vi "svl_Peak Resampled Level (N Ch).vi"(8 "error in (no error)":errorcluster, 9 "processing state":T1(ring), 11 "scaled even angle signals [EU]":T2(array[cluster]) {"even angle signal" format="%.2f"; "dr" format="%.2f"; "r0" format="%.2f"}) -> (0 "error out":errorcluster, 3 "peak levels":dbl[](array[numeric]) format="%.2f")   [LabVIEW 2017]
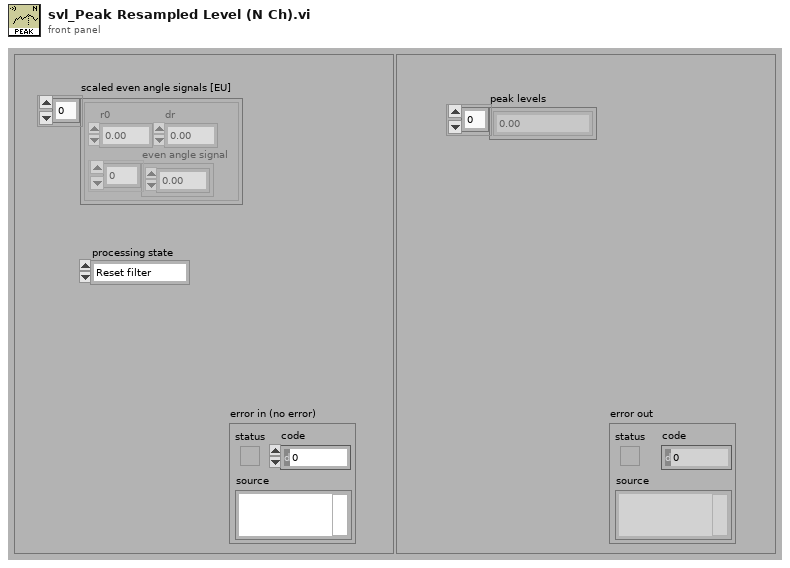
[diagram p1: front panel]
types:
  T1 = enum16{"Reset filter", "Restart averaging", "Continue processing"}
  T2 = cluster{"r0":dbl, "dr":dbl, "even angle signal":dbl[]}[]
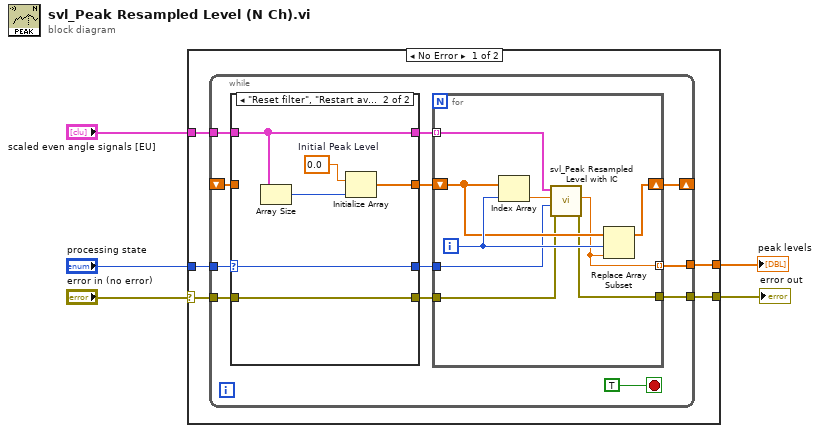
[diagram p0: block diagram]
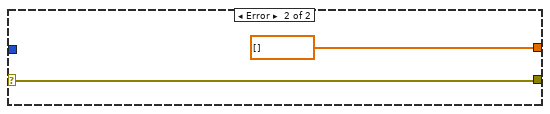
[diagram p3: hidden frame]
diagram:
  n1 = case shown="No Error" "error in (no error)" {
    selector: "error in (no error)" -> [w7 w43]
    tunnel: "processing state" -> [w10 _]
    tunnel: "scaled even angle signals [EU]" -> [w9 _]
    tunnel: [w8 dbl[] []] -> w3
    tunnel: [w6 w43] -> w1
    frame No Error {
      n2 = while {
        tunnel: [w13] -> w6
        tunnel: w7 -> [w12]
        tunnel: [w16] -> w8
        shift-left: _ -> [w18]
        shift-right: [w21] -> _
        tunnel: w9 -> [w15]
        tunnel: w10 -> [w20]
        stop <- TRUE stop-if-true
        n3 = case shown="\"Reset filter\", \"Restart averaging\"" w20 {
          selector: w20 -> [w26 w32]
          tunnel: [w26 w32] -> w19
          tunnel: w18 -> [w25 _]
          tunnel: [w25 w31] -> w17
          tunnel: w15 -> [w24 w30]
          tunnel: [w24 w30] -> w14
          tunnel: w12 -> [w23 w29]
          tunnel: [w23 w29] -> w11
          frame "Continue processing", Default {
          }
          frame "Reset filter", "Restart averaging" {
            w28 = 0.0  # Initial Peak Level
            n4 = Array Size(array=w30) -> (size(s)=w27:i32)
            n5 = Initialize Array(w28, w27) -> (w31:dbl[])
          }
        }
        n6 = for {
          tunnel: w14 -> [w33] mode=indexing
          shift-right: [w41] -> w21
          shift-left: w17 -> [w39]
          tunnel: [w35] -> w16 mode=indexing
          tunnel: w19 -> [w34]
          tunnel: w11 -> [w38]
          tunnel: [w37] -> w13
          i -> [w40]
          n7 = Index Array(array=w39, index=w40) -> (element=w36:dbl)
          n8 = call <vilib>:"svl_Peak Resampled Level with IC.vi"("error in (no error)"=w38, "processing state"=w34, "initial soundLevel"=w36, "even angle signal"=w33) -> ("error out"=w37:errorcluster, "final soundLevel"=w35:dbl)  [unwired: 6 in]
          n9 = Replace Array Subset(array=w39, new element=w35, index=w40) -> (w41:dbl[])
        }
      }
    }
    frame Error {
    }
  }
  "peak levels" <- w3
  "error out" <- w1
